vi "Copy Template UIP.vi"(11 "Dest Path":path) -> (0 "Error Out":errorcluster, 3 "Template Path":path)   [LabVIEW 2020, in "UIM.lvlib" / "UIM.lvclass"]
uses:
  UIM.lvclass
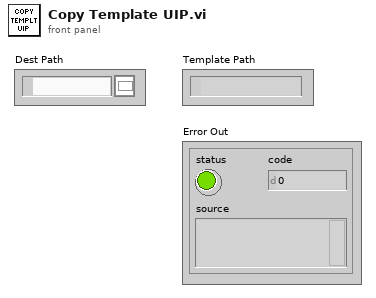
[diagram p1: front panel]
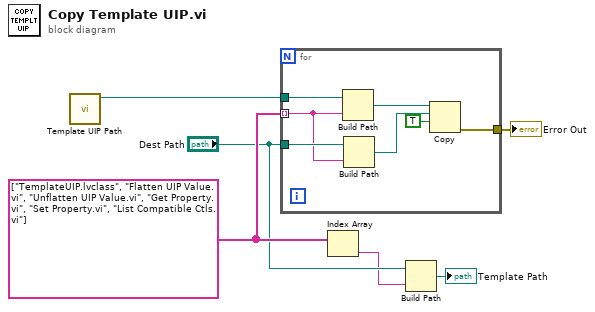
[diagram p0: block diagram]
diagram:
  w5 = string[] ["TemplateUIP.lvclass", "Flatten UIP Value.vi", "Unflatten UIP Value.vi", "Get Property.vi", "Set Property.vi", "List Compatible Ctls.vi"]
  n1 = call "Template UIP Path.vi"() -> ("Template UIP Path"=w6:path)  [unwired: 11 in]
  n2 = for {
    tunnel: w6 -> [w13]
    tunnel: w5 -> [w11] mode=indexing
    tunnel: "Dest Path" -> [w12]
    tunnel: [w7] -> w1
    n3 = Build Path(base path=w13, name or relative path=w11) -> (appended path=w10:path)
    n4 = Build Path(base path=w12, name or relative path=w11) -> (appended path=w9:path)
    n5 = Copy(9:TRUE ("overwrite (F)"), 10:w9, 11:w10) -> (0:w7:errorcluster)  [unwired: 2 in, 2 out]
  }
  "Error Out" <- w1
  n6 = Index Array(array=w5) -> (element=w3:string)  [unwired: 1 in]
  n7 = Build Path(base path="Dest Path", name or relative path=w3) -> (appended path=→"Template Path":path)
